vi "Format VI Info Image Structure.vi"(4 "Max Height (50 pixels)":i16=50, 5 "Wrap with Expand? (F)":bool, 6 "Max Width (500 pixels)":i16=500, 7 "Remove Library Name? (F)":bool, 8 "Error in":errorcluster caption="Error in (no error)", 9 "Image Type":T1, 10 "VI Info":T2, 11 "VIDoc Printer - Confluence In":refnum<class "VIDoc Printer - Confluence.lvclass">) -> (0 "Error out":errorcluster, 1 "Image Created?":bool, 2 "Image Structure Text":string, 3 "VIDoc Printer - Confluence Out":refnum<class "VIDoc Printer - Confluence.lvclass">)   [LabVIEW 2023, in "VIDoc Printer - Confluence.lvlib" / "VIDoc Printer - Confluence.lvclass"]
uses:
  VIDoc Printer - Confluence.lvclass
  Parsing/TypeDefs/Method Spec Cluster.ctl
  Parsing/TypeDefs/VI Type Extended Enum.ctl
  <vilib>/picture/picture.llb/imagedata.ctl
  Parsing/TypeDefs/Class Dispatch Type Enum.ctl
  Parsing/TypeDefs/Controls Info Cluster.ctl
  <vilib>/Utility/miscctls.llb/LVKeyTypeDef.ctl
  <vilib>/Utility/miscctls.llb/LVPointTypeDef.ctl
  Parsing/SubVIs/Structure Reporter/Tree Cluster.ctl
  Types/VI Info Image Types.ctl
  VIDoc Printer - Confluence.lvclass/VIDoc Printer - Confluence.ctl
  Accessors/Get Temporary Image Directory+.vi
  <vilib>/Utility/libraryn.llb/Create Directory Recursive.vi
  Printer/VIDoc Printer.lvclass
  Confluence Formatting/Confluence Formatting.lvlib
  Parsing/VIDoc Parsing.lvlib
  Parsing/SubVIs/Structure Reporter/Structure Reporter.lvlib
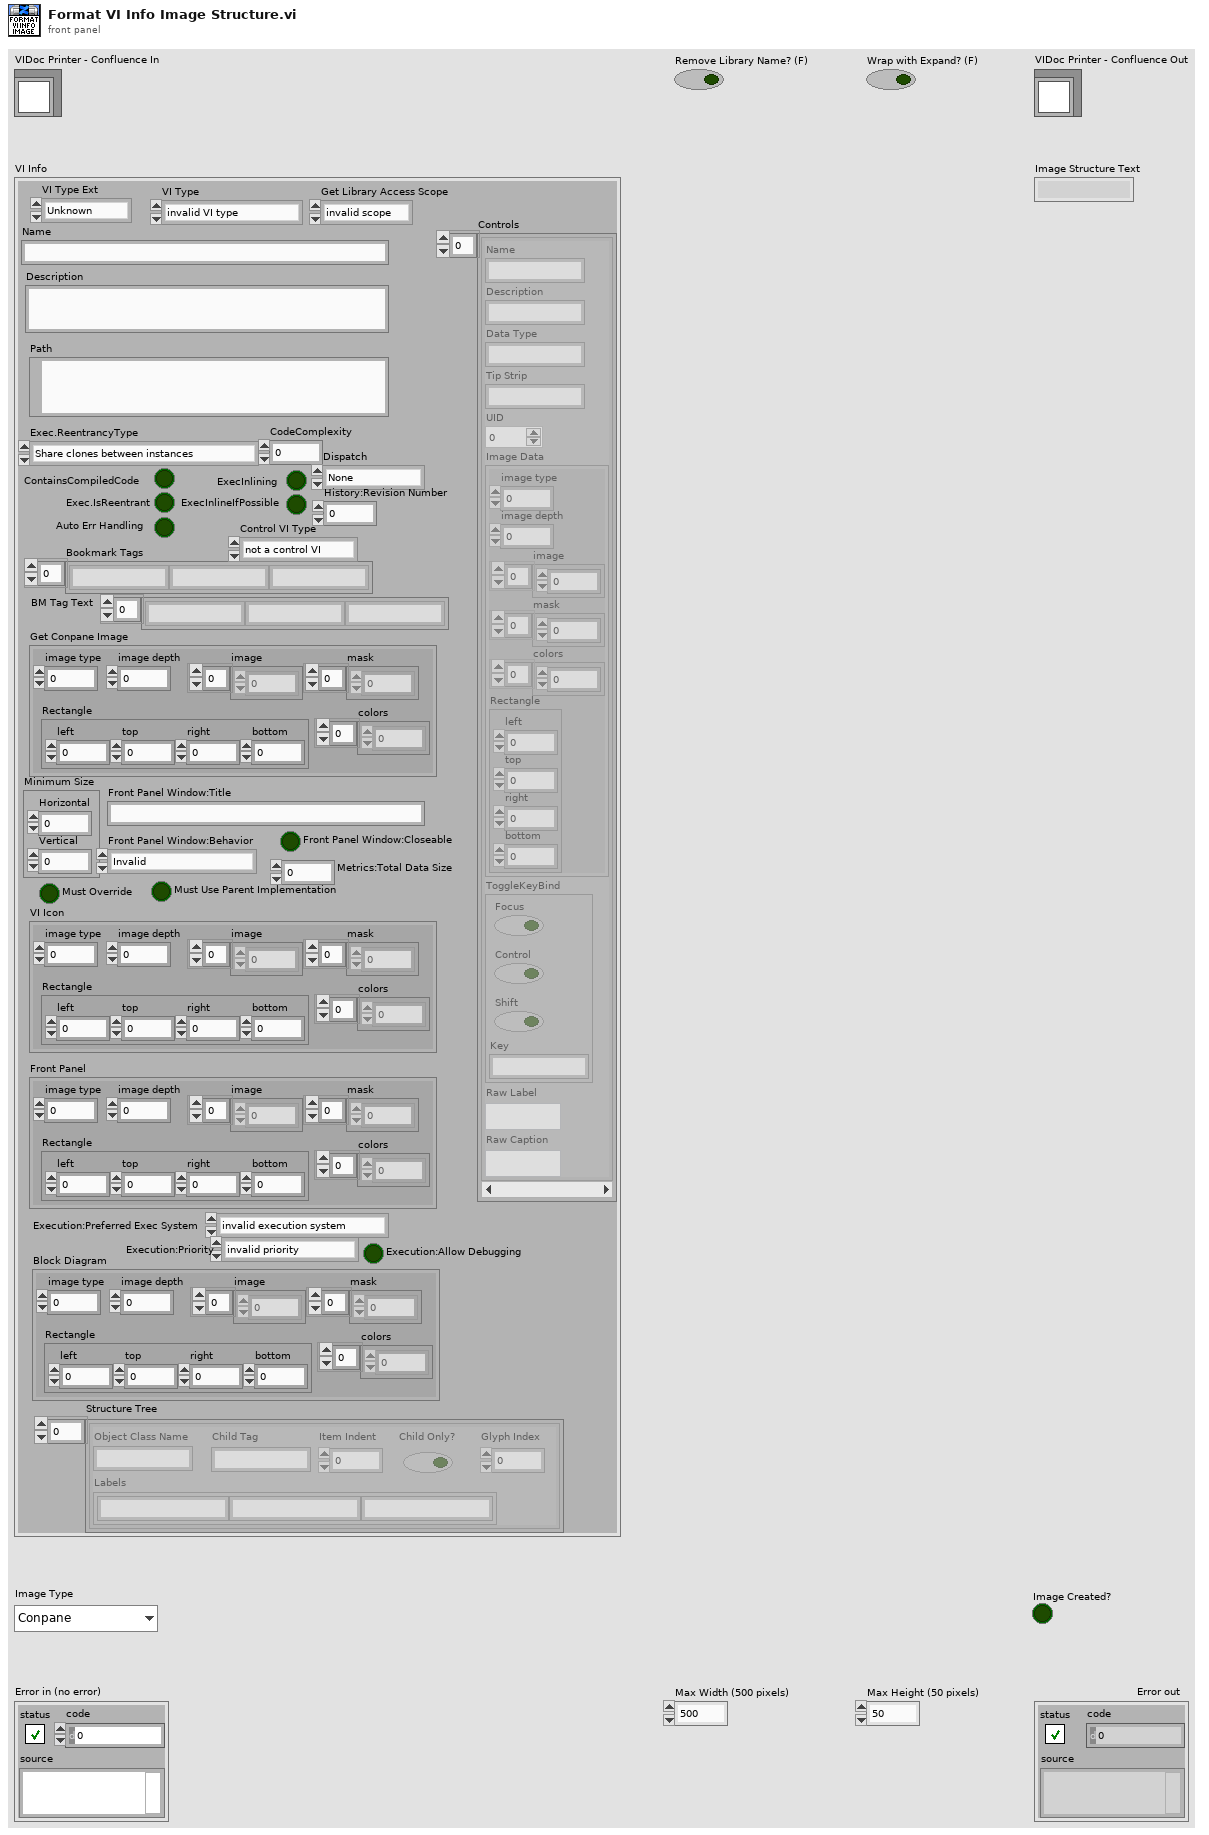
[diagram p1: front panel]
types:
  T1 = typedef "VIDoc Printer - Confluence.lvlib/VIDoc Printer - Confluence.lvclass/VI Info Image Types.ctl" = enum16{"Conpane", "FP", "BD", "Icon"}
  T2 = typedef "VIDoc Parsing.lvlib/Method Spec Cluster.ctl" = cluster{"VI Type Ext":T3, "Name":string, "Path":path, "Get Conpane Image":T4, "Description":string, "Get Library Access Scope":enum32{"invalid scope", "public", "private", "protected", "community"}, "Dispatch":T5, "ContainsCompiledCode":bool, "Exec.IsReentrant":bool, "Exec.ReentrancyType":enum16{"Share clones between instances", "Preallocate clone for each instance"}, "ExecInlining":bool, "ExecInlineIfPossible":bool, "Auto Err Handling":bool, "CodeComplexity":sgl, "Bookmark Tags":string[], "Control VI Type":enum32{"not a control VI", "control", "typedef", "strict typedef"}, "Controls":T6[], "VI Type":enum32{"invalid VI type", "Standard VI", "Control VI", "Global VI", "Polymorphic VI", "Configuration VI", "SubSystem", "Facade VI", "Method VI", "Statechart Diagram VI"}, "Minimum Size":T8, "Front Panel Window:Title":string, "Front Panel Window:Behavior":enum32{"Invalid", "Default", "Floating", "Floating/Auto-Hide", "Modal"}, "Front Panel Window:Closeable":bool, "Must Override":bool, "Must Use Parent Implementation":bool, "VI Icon":T4, "Front Panel":T4, "History:Revision Number":u32, "Metrics:Total Data Size":u32, "Execution:Allow Debugging":bool, "Execution:Preferred Exec System":enum32{"invalid execution system", "user interface", "standard", "instrument i/o", "data acquisition", "other 1", "other 2", "same as caller"}, "Execution:Priority":enum32{"invalid priority", "background priority", "normal priority", "above normal priority", "high priority", "time critical priority", "subroutine"}, "BM Tag Text":string[], "Block Diagram":T4, "Structure Tree":T9[]}
  T3 = typedef "VIDoc Parsing.lvlib/VI Type Extended Enum.ctl" = enum16{"Unknown", "Class Method", "Class Accessor Get", "Class Accessor Set", "Class Control", "Library Method", "Library Control", "VI", "Control"}
  T4 = typedef "imagedata.ctl" = cluster{"image type":i32, "image depth":i32, "image":u8[], "mask":u8[], "colors":u32[], "Rectangle":cluster{"left":i16, "top":i16, "right":i16, "bottom":i16}}
  T5 = typedef "VIDoc Parsing.lvlib/Class Dispatch Type Enum.ctl" = enum16{"None", "Static", "Dynamic"}
  T6 = typedef "VIDoc Parsing.lvlib/Controls Info Cluster.ctl" = cluster{"Name":string, "Description":string, "Data Type":string, "Tip Strip":string, "UID":i32, "Image Data":T4, "ToggleKeyBind":T7, "Raw Label":string, "Raw Caption":string}
  T7 = typedef "LVKeyTypeDef.ctl" = cluster{"Focus":bool, "Control":bool, "Shift":bool, "Key":string}
  T8 = typedef "LVPointTypeDef.ctl" = cluster{"Horizontal":i16, "Vertical":i16}
  T9 = typedef "VIDoc Parsing.lvlib/Structure Reporter.lvlib/Tree Cluster.ctl" = cluster{"Object Class Name":string, "Labels":string[], "Child Tag":string, "Item Indent":i32, "Child Only?":bool, "Glyph Index":i32}
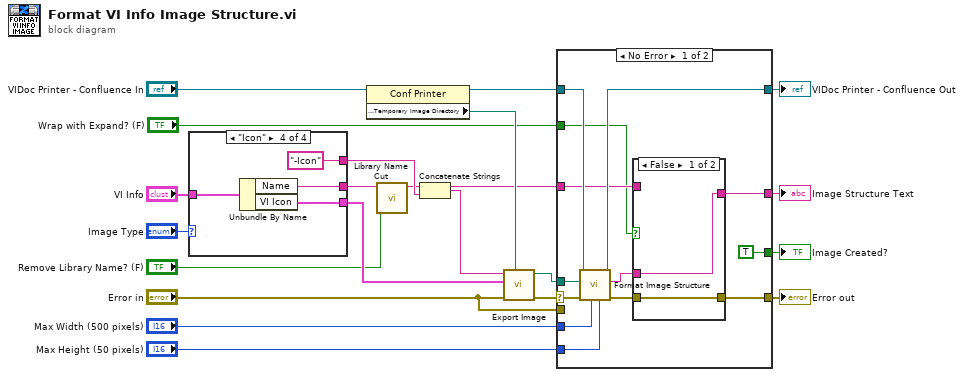
[diagram p0: block diagram]
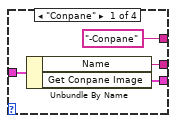
[diagram p2: hidden frame]
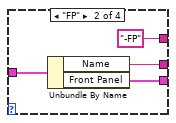
[diagram p3: hidden frame]
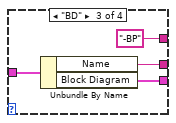
[diagram p4: hidden frame]
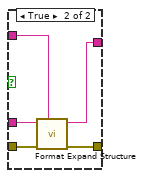
[diagram p5: hidden frame]
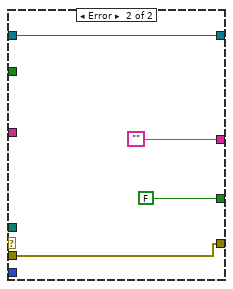
[diagram p6: hidden frame]
diagram:
  n1 = case shown="\"Icon\"" "Image Type" {
    tunnel: ["-Conpane" ("string") "-FP" ("string") "-BP" ("string") "-Icon" ("string")] -> w9
    tunnel: [w24 w28 w32 w36] -> w8
    tunnel: [w23 w27 w31 w35] -> w6
    tunnel: "VI Info" -> [w22 w26 w30 w34]
    frame "Conpane" {
      n2 = Unbundle By Name(w22) -> ("Name"=w24:string, "Get Conpane Image"=w23:T4)
    }
    frame "FP" {
      n3 = Unbundle By Name(w26) -> ("Name"=w28:string, "Front Panel"=w27:T4)
    }
    frame "BD" {
      n4 = Unbundle By Name(w30) -> ("Name"=w32:string, "Block Diagram"=w31:T4)
    }
    frame "Icon" {
      n5 = Unbundle By Name(w34) -> ("Name"=w36:string, "VI Icon"=w35:T4)
    }
  }
  n6 = property class="Conf Printer"(reference="VIDoc Printer - Confluence In") -> (reference out=w13:refnum<class "VIDoc Printer - Confluence.lvclass">, "Properties:Temporary Image Directory"=w12:path)  [unwired: 1 in, 1 out]
  n7 = call "Library Name Cut.vi"("Cut? (T)"="Remove Library Name? (F)", "Name in"=w8) -> ("Name out"=w2:string)  [unwired: 9 in]
  n8 = Concatenate Strings(w2, w9) -> (w7:string)
  n9 = call "Export Image.vi"("Temporary Image Directory"=w12, "Error in"="Error in", "Image Data"=w6, "Name"=w7) -> ("Error out"=w21:errorcluster, "Image Path"=w20:path)  [unwired: 6 in]
  n10 = case shown="No Error" w21 {
    selector: w21 -> [w50 _]
    tunnel: w20 -> [w49 _]
    tunnel: [w42 w61] -> w16
    tunnel: [w48 w59] -> w17
    tunnel: w13 -> [w47 w59]
    tunnel: [w40 ""] -> w15
    tunnel: [TRUE ("File Change Info Available?") FALSE ("File Change Info Available?")] -> w14
    tunnel: "Error in" -> [_ w61]
    tunnel: "Max Width (500 pixels)" -> [w45 _]
    tunnel: "Max Height (50 pixels)" -> [w44 _]
    tunnel: w2 -> [w39 _]
    tunnel: "Wrap with Expand? (F)" -> [w38 _]
    frame No Error {
      n11 = call "Format Image Structure.vi"("Max Height (50 pixels)"=w44, "Max Width (500 pixels)"=w45, "error in (no error)"=w50, "Image"=w49, "VIDoc Printer - Confluence In"=w47) -> ("error out"=w43:errorcluster, "Image Structure Text"=w41:string, "VIDoc Printer - Confluence Out"=w48:refnum<class "VIDoc Printer - Confluence.lvclass">)  [unwired: 4 in]
      n12 = case shown="False" w38 {
        tunnel: w43 -> [w52 w57]
        tunnel: [w52 w56] -> w42
        tunnel: w41 -> [w51 w55]
        tunnel: [w51 w54] -> w40
        tunnel: w39 -> [_ w53]
        frame False {
        }
        frame True {
          n13 = call "Format Expand Structure.vi"("Title (Click here to expand...)"=w53, "Error in"=w57, "Content"=w55) -> ("Error out"=w56:errorcluster, "Expand String"=w54:string)  [unwired: 7 in]
        }
      }
    }
    frame Error {
    }
  }
  "Error out" <- w16
  "VIDoc Printer - Confluence Out" <- w17
  "Image Structure Text" <- w15
  "Image Created?" <- w14
